vi "getStatus.vi"(8 "error in (no error)":errorcluster, 10 "MonoClientCommunicator in":refnum<class "MonoClientCommunicator.lvclass">, 11 "MonoHeartbeat in":refnum<class "MonoHeartbeat.lvclass">) -> (0 "error out":errorcluster, 1 "DeviceStatus":T1, 2 "MonoClientCommunicator out":refnum<class "MonoClientCommunicator.lvclass">, 3 "MonoHeartbeat out":refnum<class "MonoHeartbeat.lvclass">, 4 "newValue":bool)   [LabVIEW 2016, in "MonoHeartbeat.lvclass"]
uses:
  MonoHeartbeat.lvclass
  MonoClient/MonoClientCommunicator.lvclass
  Typedefs/DeviceStatus.ctl
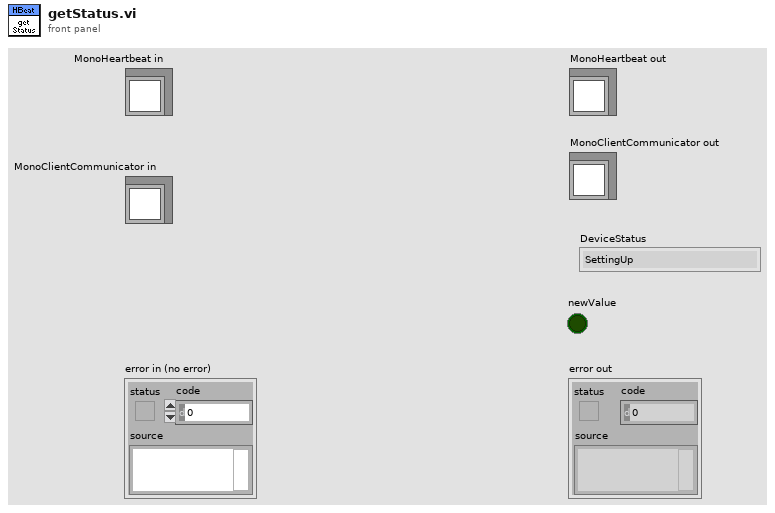
[diagram p1: front panel]
types:
  T1 = typedef "DeviceStatus.ctl" = enum16{"SettingUp", "Ready", "Offline", "Fault"}
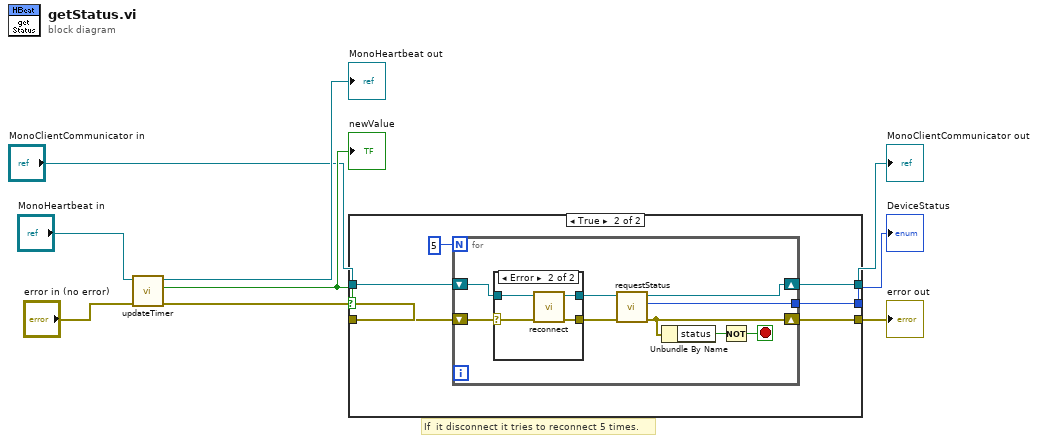
[diagram p0: block diagram]
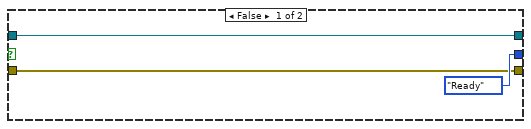
[diagram p2: hidden frame]
diagram:
  # "If  it disconnect it tries to reconnect 5 times."
  n1 = call "updateTimer.vi"("error in (no error)"="error in (no error)", "MonoHeartbeat in"="MonoHeartbeat in") -> ("error out"=w4:errorcluster, "getStatus?"=w3:bool, "MonoHeartbeat out"=→"MonoHeartbeat out":refnum<class "MonoHeartbeat.lvclass">)  [unwired: 7 in]
  "newValue" <- w3
  n2 = case shown="True" w3 {
    tunnel: [w10 w18] -> w9
    tunnel: "MonoClientCommunicator in" -> [w12 w17]
    tunnel: [w12 w16] -> w8
    tunnel: w4 -> [w10 w15]
    tunnel: [DeviceStatus."Ready" ("DeviceStatus") w14] -> w2
    frame False {
    }
    frame True {
      n3 = for {
        N: 5 -> [_]
        tunnel: [w26] -> w14
        shift-right: [w25] -> w16
        shift-left: w17 -> [w21]
        shift-right: [w19] -> w18
        shift-left: w15 -> [w20]
        stop <- w27 stop-if-true
        n4 = case shown="Error" w20 {
          selector: w20 -> [w28 w30]
          tunnel: [w28 w31] -> w24
          tunnel: w21 -> [w29 w33]
          tunnel: [w29 w32] -> w23
          frame No Error {
          }
          frame Error {
            n5 = call "reconnect.vi"("error in (no error)"=w30, "MonoClientCommunicator in"=w33) -> ("error out"=w31:errorcluster, "MonoClientCommunicator out"=w32:refnum<class "MonoClientCommunicator.lvclass">)  [unwired: 8 in]
          }
        }
        n6 = call "requestStatus.vi"("error in (no error)"=w24, "MonoClientCommunicator in"=w23) -> ("error out"=w19:errorcluster, "DeviceStatus"=w26:T1, "MonoClientCommunicator out"=w25:refnum<class "MonoClientCommunicator.lvclass">)  [unwired: 7 in]
        n7 = Unbundle By Name(w19) -> ("status"=w22:bool)
        n8 = Not(x=w22) -> (.not. x?=w27:bool)
      }
    }
  }
  "error out" <- w9
  "MonoClientCommunicator out" <- w8
  "DeviceStatus" <- w2
